vi "Database - Remove Entry.vi"(0 "reference in":refnum<class "Database_UUT.lvclass">, 9 "Part Number":string, 11 "error in (no error)":errorcluster) -> (4 "reference out":refnum<class "Database_UUT.lvclass">, 15 "error out":errorcluster)   [LabVIEW 2017, in "Database_UUT.lvclass"]
uses:
  Database_UUT.lvclass
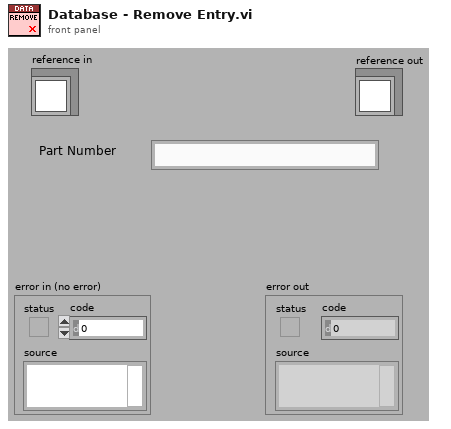
[diagram p1: front panel]
types:
  T1 = enum16{"open", "open or create", "create or replace", "create", "open (read-only)"}
  T2 = typedef "Database_UUT.lvclass/ObjectAttributes.ctl" = cluster{"Filepath to Database":path}
  T3 = cluster{"property values":variant[], "property names":string[], string}
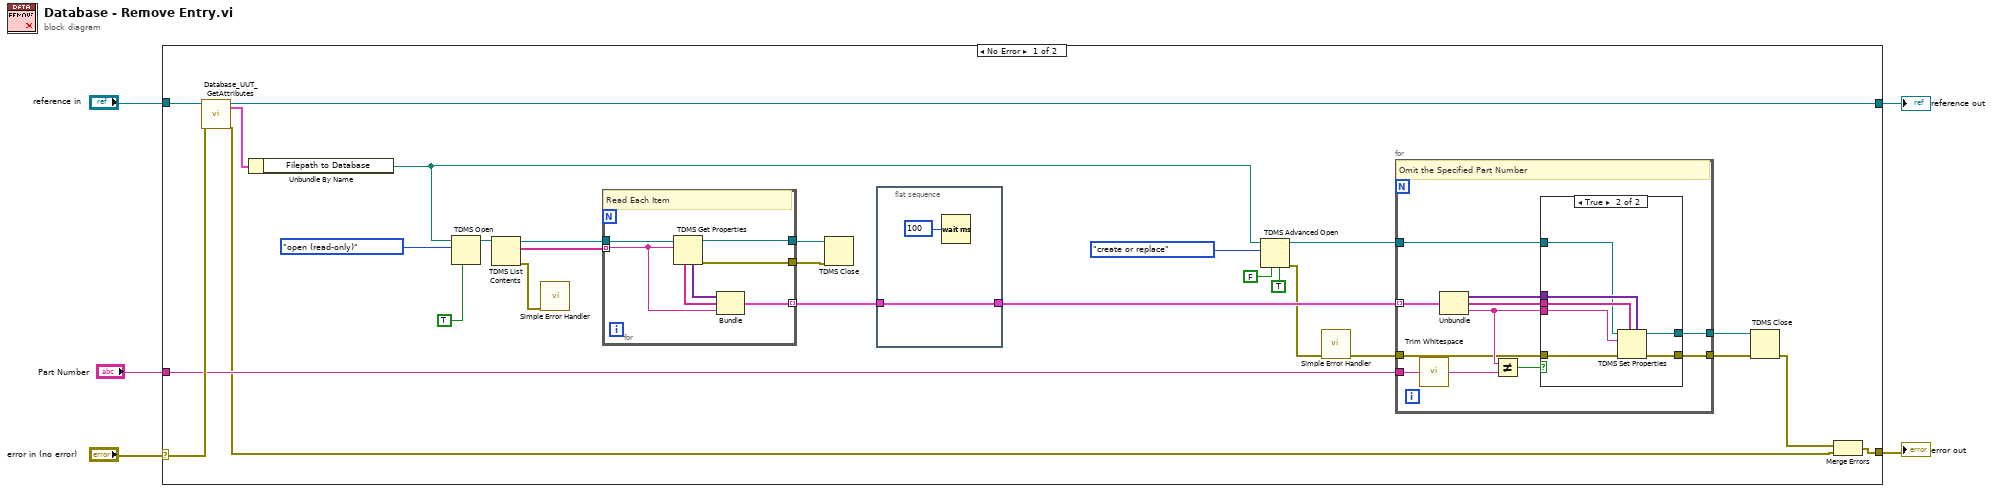
[diagram p0: block diagram]
diagram:
  n1 = case shown="No Error" "error in (no error)" {
    selector: "error in (no error)" -> [w31 w62]
    tunnel: [w19 w62] -> w4
    tunnel: [w29 w61] -> w2
    tunnel: "reference in" -> [w32 w61]
    tunnel: "Part Number" -> [w26 _]
    frame No Error {
      n2 = call "Database_UUT_GetAttributes.vi"("reference in"=w32, "error in (no error)"=w31) -> ("reference out"=w29:refnum<class "Database_UUT.lvclass">, "Data"=w30:T2, "error out"=w18:errorcluster)  [unwired: 14 in, 1 out]
      n3 = Unbundle By Name(w30) -> ("Filepath to Database"=w15:path)
      n4 = TDMS Open(6:TRUE ("enable asynchronous? (T)"), 10:T1."open (read-only)" ("operation (0:open)"), 11:w15) -> (3:w27:refnum<k34>)  [unwired: 4 in, 1 out]
      n5 = TDMS List Contents(7:w27) -> (0:w13:errorcluster, 2:w25:string[], 3:w24:refnum<k34>)  [unwired: 2 in, 1 out]
      n6 = call <vilib>:"Simple Error Handler.vi"("error in (no error)"=w13) -> ()  [unwired: 4 in, 5 out]
      n7 = for {
        tunnel: w25 -> [w36] mode=indexing
        tunnel: w24 -> [w41]
        tunnel: [w39] -> w23
        tunnel: [w40] -> w17 mode=indexing
        tunnel: [w35] -> w6
        # "Read Each Item"
        n8 = TDMS Get Properties(10:w36, 11:w41) -> (0:w35:errorcluster, 3:w39:refnum<k34>, 4:w38:variant[], 6:w37:string[])  [unwired: 4 in, 2 out]
        n9 = Bundle("property values"=w38, "property names"=w37, w36) -> (w40:T3)  [unwired: 1 in]
      }
      n10 = TDMS Close(8:w6, 11:w23) -> ()  [unwired: 2 out]
      n11 = flat-sequence {
        tunnel: w17 -> [w34]
        tunnel: [w34] -> w16
        frame #0 {
          n12 = Wait (ms)(milliseconds to wait=u32 100) -> ()  [unwired: 1 out]
        }
      }
      n13 = TDMS Advanced Open(4:TRUE ("enable asynchronous? (T)"), 6:FALSE ("disable buffering? (T)"), 10:T1."create or replace" ("operation (0:open)"), 11:w15) -> (0:w12:errorcluster, 3:w21:refnum<k34>)  [unwired: 1 in, 1 out]
      n14 = call <vilib>:"Simple Error Handler.vi"("error in (no error)"=w12) -> ("error out"=w7:errorcluster)  [unwired: 4 in, 4 out]
      n15 = for {
        tunnel: w26 -> [w52]
        tunnel: w16 -> [w49] mode=indexing
        tunnel: w21 -> [w45]
        tunnel: [w44] -> w20
        tunnel: [w43] -> w9
        tunnel: w7 -> [w42]
        # "Omit the Specified Part Number"
        n16 = call <vilib>:"Trim Whitespace.vi"("string"=w52) -> ("trimmed string"=w51:string)  [unwired: 1 in]
        n17 = Unbundle(w49) -> ("property values"=w46:variant[], "property names"=w47:string[], w48:string)
        n18 = Not Equal?(x=w48, y=w51) -> (x != y?=w50:bool)
        n19 = case shown="True" w50 {
          tunnel: w48 -> [_ w60]
          tunnel: w47 -> [_ w59]
          tunnel: w46 -> [_ w58]
          tunnel: w45 -> [w53 w57]
          tunnel: [w53 w56] -> w44
          tunnel: [_ w55] -> w43
          tunnel: w42 -> [_ w54]
          frame False {
          }
          frame True {
            n20 = TDMS Set Properties(5:w58, 7:w59, 8:w54, 10:w60, 11:w57) -> (0:w55:errorcluster, 3:w56:refnum<k34>)  [unwired: 1 in, 2 out]
          }
        }
      }
      n21 = TDMS Close(8:w9, 11:w20) -> (0:w8:errorcluster)  [unwired: 1 out]
      n22 = Merge Errors(w8, w18) -> (w19:errorcluster)
    }
    frame Error {
    }
  }
  "error out" <- w4
  "reference out" <- w2
